vi "subSave_AcquireLightInfomation.vi"(1 "AO (V)":dbl[](array[slide])=[0.0, 0.0, 0.0, 0.0, 0.0] min=0.0 max=5.0 step=0.01 scale=0.0..5.0 scale format="%#1.2f", 2 "DO":bool[](array[boolean])=[FALSE, FALSE, FALSE, FALSE, FALSE, FALSE, FALSE], 3 "LED":bool) -> (0 "Text out":string)   [LabVIEW 2015]
panel:
  # "Global"
  # "637"
  # "561"
  # "532"
  # "488"
  # "405"
  # "Red"
  # "DO"
  # "AO"
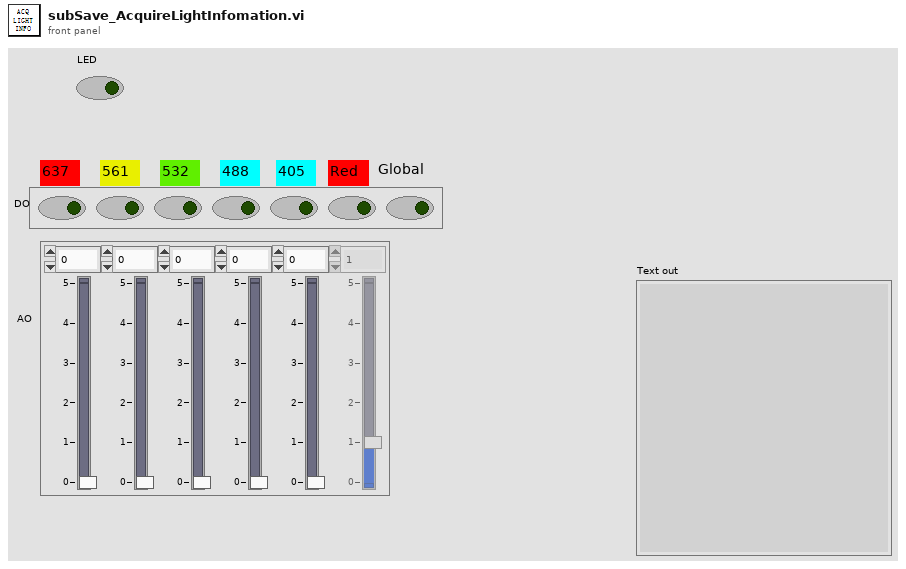
[diagram p1: front panel]
types:
  T1 = cluster{"DO[0]":bool, "DO[1]":bool, "DO[2]":bool, "DO[3]":bool, "DO[4]":bool, "DO[5]":bool, "DO[6]":bool, "DO[7]":bool, "DO[8]":bool}
  T2 = cluster{"AO (V)[0]":dbl, "AO (V)[1]":dbl, "AO (V)[2]":dbl, "AO (V)[3]":dbl, "AO (V)[4]":dbl, "AO (V)[5]":dbl, "AO (V)[6]":dbl, "AO (V)[7]":dbl, "AO (V)[8]":dbl}
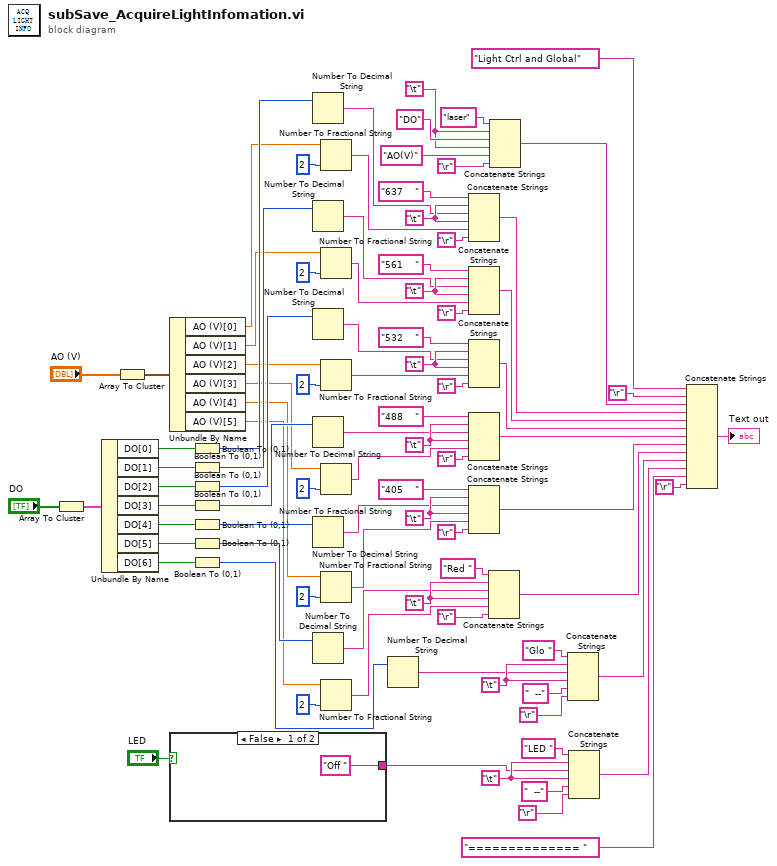
[diagram p0: block diagram]
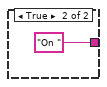
[diagram p2: hidden frame]
diagram:
  w11 = "\t"
  w28 = "\t"
  w33 = "\t"
  w39 = "\t"
  w45 = "\t"
  w51 = "\t"
  w57 = "\t"
  w64 = "\t"
  w88 = "\t"
  n1 = Array To Cluster(array="DO") -> (cluster=w13:T1)
  n2 = Unbundle By Name(w13) -> ("DO[0]"=w84:bool, "DO[1]"=w76:bool, "DO[2]"=w75:bool, "DO[3]"=w74:bool, "DO[4]"=w73:bool, "DO[5]"=w72:bool, "DO[6]"=w71:bool)
  n3 = Array To Cluster(array="AO (V)") -> (cluster=w85:T2)
  n4 = Unbundle By Name(w85) -> ("AO (V)[0]"=w70:dbl, "AO (V)[1]"=w69:dbl, "AO (V)[2]"=w68:dbl, "AO (V)[3]"=w67:dbl, "AO (V)[4]"=w66:dbl, "AO (V)[5]"=w7:dbl)
  n5 = case shown="False" "LED" {
    tunnel: ["Off " ("string") "On " ("string")] -> w4
    frame False {
    }
    frame True {
    }
  }
  n6 = Boolean To (0,1)(Boolean=w84) -> (0, 1=w81:i16)
  n7 = Boolean To (0,1)(Boolean=w76) -> (0, 1=w80:i16)
  n8 = Boolean To (0,1)(Boolean=w75) -> (0, 1=w83:i16)
  n9 = Boolean To (0,1)(Boolean=w74) -> (0, 1=w82:i16)
  n10 = Boolean To (0,1)(Boolean=w73) -> (0, 1=w79:i16)
  n11 = Boolean To (0,1)(Boolean=w72) -> (0, 1=w78:i16)
  n12 = Boolean To (0,1)(Boolean=w71) -> (0, 1=w77:i16)
  n13 = Number To Decimal String(number=w81) -> (decimal integer string=w62:string)  [unwired: 1 in]
  n14 = Number To Decimal String(number=w80) -> (decimal integer string=w55:string)  [unwired: 1 in]
  n15 = Number To Decimal String(number=w83) -> (decimal integer string=w49:string)  [unwired: 1 in]
  n16 = Number To Decimal String(number=w82) -> (decimal integer string=w43:string)  [unwired: 1 in]
  n17 = Number To Decimal String(number=w79) -> (decimal integer string=w37:string)  [unwired: 1 in]
  n18 = Number To Decimal String(number=w78) -> (decimal integer string=w31:string)  [unwired: 1 in]
  n19 = Number To Fractional String(number=w70, precision (6)=i16 2) -> (F-format string=w61:string)  [unwired: 2 in]
  n20 = Number To Fractional String(number=w69, precision (6)=i16 2) -> (F-format string=w54:string)  [unwired: 2 in]
  n21 = Number To Fractional String(number=w68, precision (6)=i16 2) -> (F-format string=w48:string)  [unwired: 2 in]
  n22 = Number To Fractional String(number=w67, precision (6)=i16 2) -> (F-format string=w42:string)  [unwired: 2 in]
  n23 = Number To Fractional String(number=w66, precision (6)=i16 2) -> (F-format string=w36:string)  [unwired: 2 in]
  n24 = Number To Fractional String(number=w7, precision (6)=i16 2) -> (F-format string=w6:string)  [unwired: 2 in]
  n25 = Number To Decimal String(number=w77) -> (decimal integer string=w26:string)  [unwired: 1 in]
  n26 = Concatenate Strings("637    " ("string"), w64, w62, w64, w61, "\r") -> (w59:string)
  n27 = Concatenate Strings("561    " ("string"), w57, w55, w57, w54, "\r") -> (w53:string)
  n28 = Concatenate Strings("532    " ("string"), w51, w49, w51, w48, "\r") -> (w47:string)
  n29 = Concatenate Strings("488    " ("string"), w45, w43, w45, w42, "\r") -> (w41:string)
  n30 = Concatenate Strings("405    " ("string"), w39, w37, w39, w36, "\r") -> (w35:string)
  n31 = Concatenate Strings("Red " ("string"), w33, w31, w33, w6, "\r") -> (w25:string)
  n32 = Concatenate Strings("laser" ("string"), w88, "DO" ("string"), w88, "AO(V)" ("string"), "\r") -> (w60:string)
  n33 = Concatenate Strings("Glo " ("string"), w28, w26, w28, "  --" ("string"), "\r") -> (w24:string)
  n34 = Concatenate Strings("LED " ("string"), w11, w4, w11, "  --" ("string"), "\r") -> (w2:string)
  n35 = Concatenate Strings("Light Ctrl and Global" ("string"), "\r", w60, w59, w53, w47, w41, w35, w25, w24, w2, "============== " ("string"), "\r") -> (→"Text out":string)
